vi "CRYCal Harmonics.vi"(0 "HT Option":bool[](array[boolean]), 1 "x":dbl[](array[numeric]), 2 "z":dbl[](array[numeric]), 3 "Index":i32, 5 "Method":u16, 7 "Harmonic":dbl[](array[numeric]), 9 "Freq resp curves":dbl[][](array[numeric]), 11 "Total Noise":dbl[](array[numeric]), 12 "Fs":dbl format="%.2f", 13 "max value1":dbl, 14 "max value2":dbl) -> (4 "Harmonic Track Out":T1(array[cluster]))   [LabVIEW 2013]
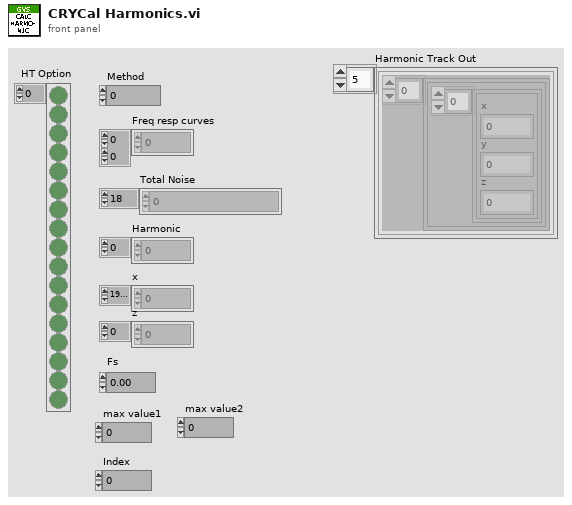
[diagram p1: front panel]
types:
  T1 = cluster{cluster{cluster{"x":dbl, "y":dbl, "z":dbl}[]}[]}[]
  T2 = cluster{"Freq resp curves clipped":cluster{cluster{"x":dbl, "y":dbl, "z":dbl}[]}[]}[]
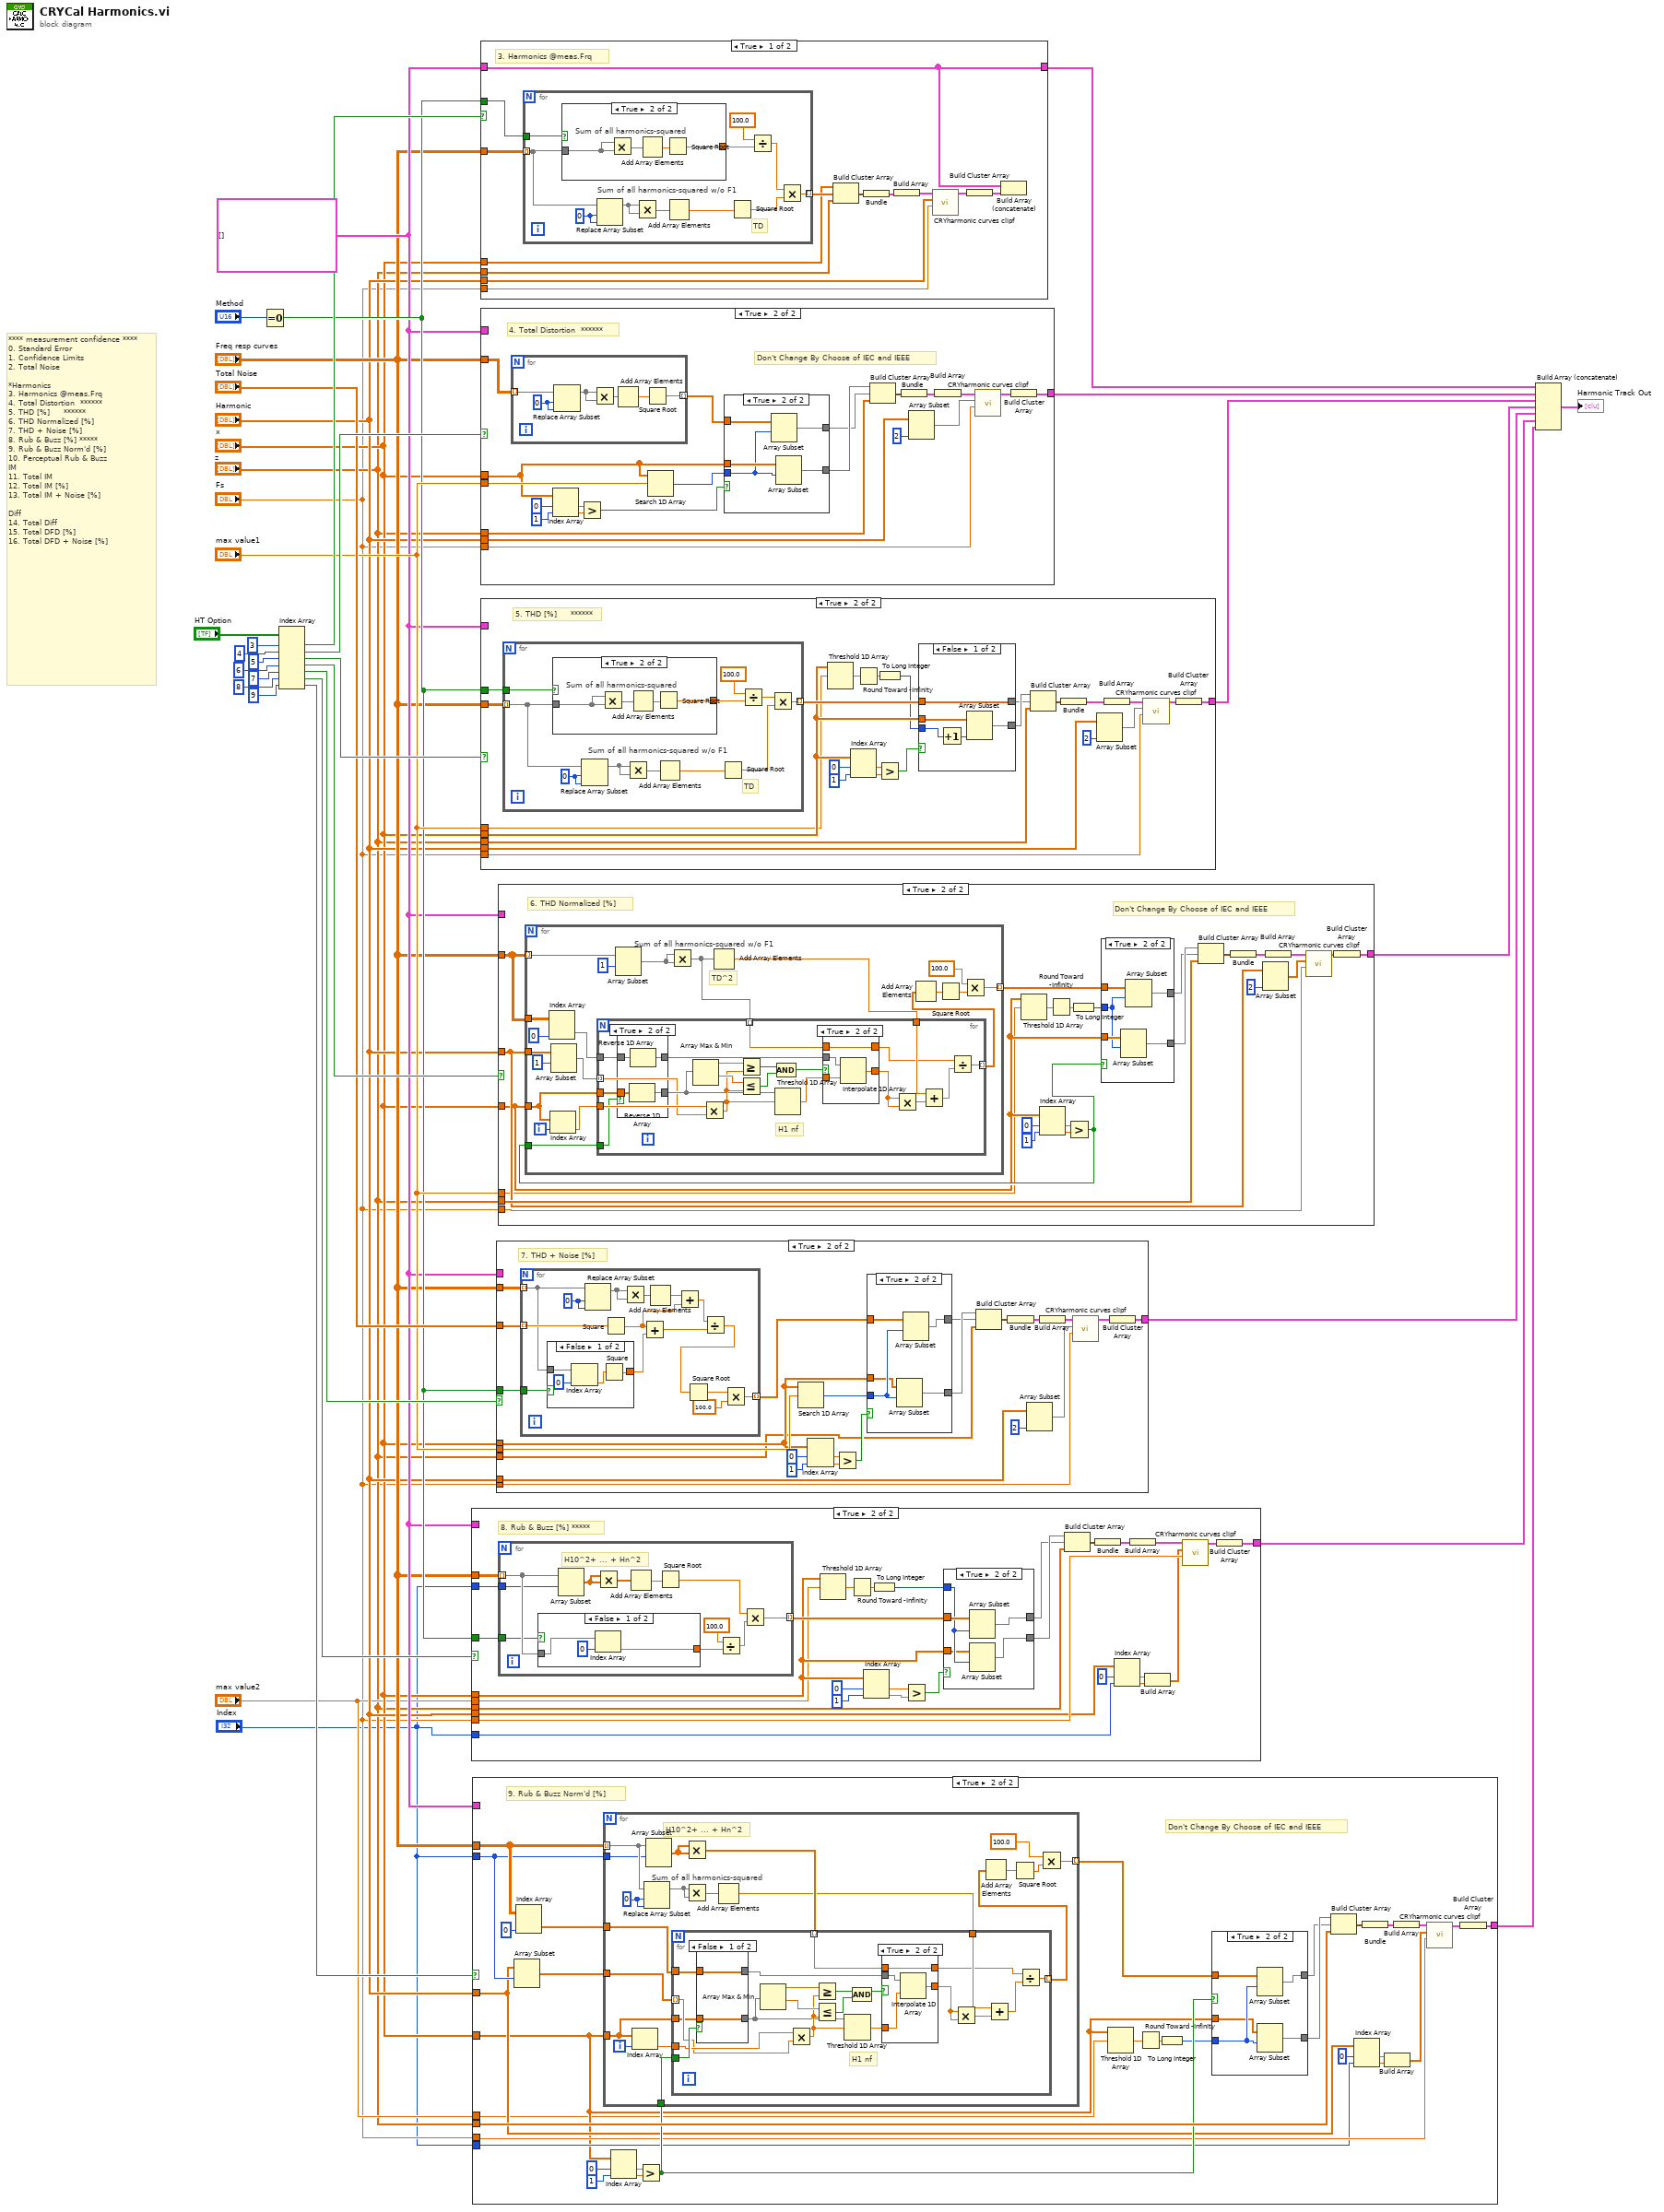
[diagram p0: block diagram]
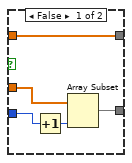
[diagram p3: hidden frame]
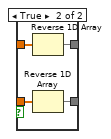
[diagram p4: hidden frame]
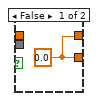
[diagram p5: hidden frame]
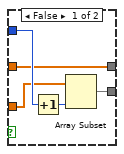
[diagram p7: hidden frame]
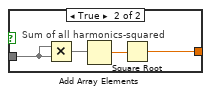
[diagram p8: hidden frame]
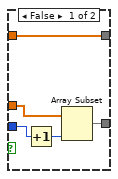
[diagram p10: hidden frame]
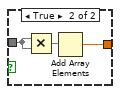
[diagram p11: hidden frame]
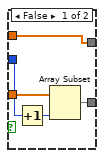
[diagram p13: hidden frame]
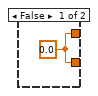
[diagram p15: hidden frame]
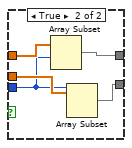
[diagram p17: hidden frame]
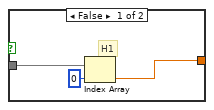
[diagram p18: hidden frame]
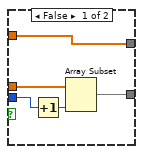
[diagram p20: hidden frame]
diagram:
  w10 = cluster{cluster{cluster[]}[]}[] []
  # "**** measurement confidence ****\n0. Standard Error\n1. Confidence Limits\n2. Total Noise\n\n*Harmonics\n3. Harmonics @meas.Frq\n4. Total Distortion  ******\n5. THD [%]     ******\n6. THD Normalized [%]\n7. THD + Noise [%]\n8. Rub & Buzz [%] *****\n9. Rub & Buzz Norm'd [%]\n10. Perceptual Rub & Buzz \nIM\n11. Total IM\n12. Total IM [%]\n13. Total IM + Noise [%]\n\nDiff\n14. Total Diff\n15. Total DFD [%]\n16. Total DFD + Noise [%]"
  n1 = Equal To 0?(x="Method") -> (x = 0?=w12:bool)
  n2 = Index Array(array="HT Option", index #1=3 ("index"), index #2=4 ("index"), index #3=5 ("index"), index #4=6 ("index"), index #5=7 ("index"), index #6=8 ("index"), index #7=9 ("index")) -> (element #1=w26:bool, element #2=w25:bool, element #3=w24:bool, element #4=w19:bool, element #5=w17:bool, element #6=w13:bool, element #7=w8:bool)
  n3 = case shown="True" w13 {
    tunnel: "Freq resp curves" -> [_ w58]
    tunnel: w12 -> [_ w57]
    tunnel: "x" -> [_ w39]
    tunnel: "max value2" -> [_ w38]
    tunnel: "Fs" -> [_ w56]
    tunnel: "z" -> [_ w55]
    tunnel: [w36 w49] -> w11
    tunnel: w10 -> [w36 _]
    tunnel: "Index" -> [_ w48]
    tunnel: "Harmonic" -> [_ w43]
    tunnel: "Index" -> [_ w42]
    frame False {
    }
    frame True {
      # "8. Rub & Buzz [%] *****"
      n4 = for {
        tunnel: [w81] -> w61 mode=indexing
        tunnel: w58 -> [w80] mode=indexing
        tunnel: w57 -> [w79]
        tunnel: w48 -> [w76]
        # "H10^2+ ... + Hn^2"
        n5 = case shown="False" w79 {
          tunnel: [w87 w92] -> w82
          tunnel: w80 -> [w88 w91]
          frame False {
            n6 = Index Array(array=w88, index=0) -> (element=w87:dbl)
          }
          frame True {
            # "Sum of all harmonics-squared"
            n7 = Multiply(x=w91, y=w91) -> (x*y=w90:dbl[])
            n8 = Add Array Elements(numeric array=w90) -> (sum=w93:dbl)
            n9 = Square Root(x=w93) -> (sqrt(x)=w92:dbl)
          }
        }
        n10 = Array Subset(array=w80, index=w76) -> (w78:dbl[])  [unwired: 1 in]
        n11 = Multiply(x=w78, y=w78) -> (x*y=w77:dbl[])
        n12 = Add Array Elements(numeric array=w77) -> (sum=w85:dbl)
        n13 = Square Root(x=w85) -> (sqrt(x)=w83:dbl)
        n14 = Divide(x=100.0, y=w82) -> (x/y=w84:dbl)
        n15 = Multiply(x=w83, y=w84) -> (x*y=w81:dbl)
      }
      n16 = Threshold 1D Array(2:w38, 3:w39) -> (0:w41:dbl)  [unwired: 1 in]
      n17 = Round Toward -Infinity(1:w41) -> (0:w40:dbl)
      n18 = Index Array(array=w39, index #1=0 ("index"), index #2=1 ("index")) -> (element #1=w52:dbl, element #2=w51:dbl)
      n19 = To Long Integer(number=w40) -> (32bit integer=w37:i32)
      n20 = Greater?(x=w52, y=w51) -> (0:w50:bool)
      n21 = case shown="True" w50 {
        tunnel: w37 -> [w70 w72]
        tunnel: [w68 w75] -> w62
        tunnel: [w67 w73] -> w60
        tunnel: w61 -> [w67 w74]
        tunnel: w39 -> [w66 w71]
        frame False {
          n22 = Increment(x=w70) -> (x+1=w69:i32)
          n23 = Array Subset(array=w66, length=w69) -> (w68:dbl[])  [unwired: 1 in]
        }
        frame True {
          n24 = Array Subset(array=w74, index=w72) -> (w73:dbl[])  [unwired: 1 in]
          n25 = Array Subset(array=w71, index=w72) -> (w75:dbl[])  [unwired: 1 in]
        }
      }
      n26 = Build Cluster Array(w62, w60, w55) -> (w64:cluster{"x":dbl, dbl, "Z":dbl}[])
      n27 = Bundle(w64) -> (w65:cluster{cluster{"x":dbl, dbl, "Z":dbl}[]})  [unwired: 1 in]
      n28 = Index Array(array=w43, index #1=0 ("Index"), index #2=w42) -> (element #1=w46:dbl, element #2=w45:dbl)
      n29 = Build Array(w65) -> (w59:cluster{cluster{"x":dbl, dbl, "Z":dbl}[]}[])
      n30 = Build Array(w46, w45) -> (w44:dbl[])
      n31 = call "CRYharmonic curves clipf.vi"("Fs"=w56, "Harmonics"=w44, "Freq resp curves"=w59) -> ("Freq resp curves clipped"=w63:cluster{cluster{"x":dbl, "y":dbl, "z":dbl}[]}[])  [unwired: 8 out]
      n32 = Build Cluster Array(w63) -> (w49:T2)
    }
  }
  n33 = case shown="True" w8 {
    tunnel: [w94 w118] -> w1
    tunnel: w10 -> [w94 _]
    tunnel: "Freq resp curves" -> [_ w104]
    tunnel: "Harmonic" -> [_ w101]
    tunnel: "x" -> [_ w97]
    tunnel: "max value2" -> [_ w96]
    tunnel: "z" -> [_ w113]
    tunnel: "Fs" -> [_ w107]
    tunnel: "Index" -> [_ w106]
    tunnel: "Index" -> [_ w102]
    frame False {
    }
    frame True {
      # "9. Rub & Buzz Norm'd [%]"
      # "Don't Change By Choose of IEC and IEEE"
      n34 = Array Subset(array=w101, index=w102) -> (w100:dbl[])  [unwired: 1 in]
      n35 = Index Array(array=w104, index (col)=0 ("disabled index (col)")) -> (element=w103:dbl[])  [unwired: 1 in]
      n36 = Index Array(array=w97, index #1=0 ("index"), index #2=1 ("index")) -> (element #1=w116:dbl, element #2=w117:dbl)
      n37 = Greater?(x=w116, y=w117) -> (0:w112:bool)
      n38 = for {
        tunnel: [w154] -> w121 mode=indexing
        tunnel: w104 -> [w142] mode=indexing
        tunnel: w97 -> [w140]
        tunnel: w112 -> [w141]
        tunnel: w102 -> [w138]
        tunnel: w103 -> [w137]
        tunnel: w100 -> [w136]
        i -> [w143]
        w145 = 0
        # "H10^2+ ... + Hn^2"
        # "Sum of all harmonics-squared"
        n39 = Index Array(array=w140, index=w143) -> (element=w153:dbl)
        n40 = Replace Array Subset(array=w142, new element=w145, index=w145) -> (w144:dbl[])
        n41 = Array Subset(array=w142, index=w138) -> (w139:dbl[])  [unwired: 1 in]
        n42 = Multiply(x=w139, y=w139) -> (x*y=w148:dbl[])
        n43 = Multiply(x=w144, y=w144) -> (x*y=w151:dbl[])
        n44 = Add Array Elements(numeric array=w151) -> (sum=w146:dbl)
        n45 = for {
          tunnel: w137 -> [w163]
          tunnel: w146 -> [w175]
          tunnel: w153 -> [w157]
          tunnel: w148 -> [w160] mode=indexing
          tunnel: [w171] -> w152 mode=indexing
          tunnel: w136 -> [w156] mode=indexing
          tunnel: w141 -> [w158]
          tunnel: w140 -> [w155]
          # "H1 nf"
          n46 = case shown="False" w158 {
            tunnel: w163 -> [w177 w178]
            tunnel: [w177 w181] -> w162
            tunnel: [w176 w180] -> w161
            tunnel: w155 -> [w176 w179]
            frame False {
            }
            frame True {
              n47 = Reverse 1D Array(array=w178) -> (reversed array=w181:dbl[])
              n48 = Reverse 1D Array(array=w179) -> (reversed array=w180:dbl[])
            }
          }
          n49 = Array Max & Min(array=w161) -> (max value=w168:dbl, min value=w167:dbl)  [unwired: 2 out]
          n50 = Multiply(x=w157, y=w156) -> (x*y=w166:dbl)
          n51 = Greater Or Equal?(x=w168, y=w166) -> (x >= y?=w169:bool)
          n52 = Less Or Equal?(x=w167, y=w166) -> (x <= y?=w164:bool)
          n53 = Threshold 1D Array(2:w166, 3:w161) -> (0:w170:dbl)  [unwired: 1 out]
          n54 = Compound Arithmetic op=AND(w169, w164) -> (w165:bool)
          n55 = case shown="True" w165 {
            tunnel: w162 -> [_ w183]
            tunnel: [w182 w184] -> w173
            tunnel: w170 -> [_ w185]
            tunnel: w160 -> [_ w186]
            tunnel: [w182 w186] -> w159
            frame False {
              w182 = 0.0 ("y")
            }
            frame True {
              n56 = Interpolate 1D Array(1:w185, 2:w183) -> (0:w184:dbl)
            }
          }
          n57 = Multiply(x=w173, y=w173) -> (x*y=w174:dbl)
          n58 = Add(x=w175, y=w174) -> (x+y=w172:dbl)
          n59 = Divide(x=w159, y=w172) -> (x/y=w171:dbl)
        }
        n60 = Add Array Elements(numeric array=w152) -> (sum=w149:dbl)
        n61 = Square Root(x=w149) -> (sqrt(x)=w147:dbl)
        n62 = Multiply(x=100.0, y=w147) -> (x*y=w154:dbl)
      }
      n63 = Threshold 1D Array(2:w96, 3:w97) -> (0:w98:dbl)  [unwired: 1 in]
      n64 = Round Toward -Infinity(1:w98) -> (0:w99:dbl)
      n65 = To Long Integer(number=w99) -> (32bit integer=w95:i32)
      n66 = case shown="True" w112 {
        tunnel: w95 -> [w130 w132]
        tunnel: [w128 w135] -> w122
        tunnel: w121 -> [w127 w134]
        tunnel: [w127 w133] -> w120
        tunnel: w97 -> [w126 w131]
        frame False {
          n67 = Increment(x=w130) -> (x+1=w129:i32)
          n68 = Array Subset(array=w126, length=w129) -> (w128:dbl[])  [unwired: 1 in]
        }
        frame True {
          n69 = Array Subset(array=w134, index=w132) -> (w133:dbl[])  [unwired: 1 in]
          n70 = Array Subset(array=w131, index=w132) -> (w135:dbl[])  [unwired: 1 in]
        }
      }
      n71 = Build Cluster Array(w122, w120, w113) -> (w124:cluster{"x":dbl, dbl, "Z":dbl}[])
      n72 = Index Array(array=w101, index #1=0 ("Index"), index #2=w106) -> (element #1=w110:dbl, element #2=w109:dbl)
      n73 = Bundle(w124) -> (w125:cluster{cluster{"x":dbl, dbl, "Z":dbl}[]})  [unwired: 1 in]
      n74 = Build Array(w110, w109) -> (w108:dbl[])
      n75 = Build Array(w125) -> (w119:cluster{cluster{"x":dbl, dbl, "Z":dbl}[]}[])
      n76 = call "CRYharmonic curves clipf.vi"("Fs"=w107, "Harmonics"=w108, "Freq resp curves"=w119) -> ("Freq resp curves clipped"=w123:cluster{cluster{"x":dbl, "y":dbl, "z":dbl}[]}[])  [unwired: 8 out]
      n77 = Build Cluster Array(w123) -> (w118:T2)
    }
  }
  n78 = case shown="True" w26 {
    tunnel: w10 -> [w192 w218]
    tunnel: "Freq resp curves" -> [w199 _]
    tunnel: [w192 w218] -> w23
    tunnel: w12 -> [w194 _]
    tunnel: "x" -> [w190 _]
    tunnel: "z" -> [w189 _]
    tunnel: "Harmonic" -> [w188 _]
    tunnel: "Fs" -> [w187 _]
    frame True {
      # "3. Harmonics @meas.Frq"
      n79 = for {
        tunnel: w199 -> [w201] mode=indexing
        tunnel: [w203] -> w198 mode=indexing
        tunnel: w194 -> [w200]
        w202 = 0
        # "TD"
        # "Sum of all harmonics-squared w/o F1"
        n80 = case shown="True" w200 {
          tunnel: [w211 w215] -> w204
          tunnel: w201 -> [w212 w214]
          frame False {
            # "H1"
            n81 = Index Array(array=w212, index=0) -> (element=w211:dbl)
          }
          frame True {
            # "Sum of all harmonics-squared"
            n82 = Multiply(x=w214, y=w214) -> (x*y=w217:dbl[])
            n83 = Add Array Elements(numeric array=w217) -> (sum=w216:dbl)
            n84 = Square Root(x=w216) -> (sqrt(x)=w215:dbl)
          }
        }
        n85 = Replace Array Subset(array=w201, new element=w202, index=w202) -> (w208:dbl[])
        n86 = Multiply(x=w208, y=w208) -> (x*y=w206:dbl[])
        n87 = Add Array Elements(numeric array=w206) -> (sum=w207:dbl)
        n88 = Square Root(x=w207) -> (sqrt(x)=w210:dbl)
        n89 = Divide(x=100.0, y=w204) -> (x/y=w205:dbl)
        n90 = Multiply(x=w205, y=w210) -> (x*y=w203:dbl)
      }
      n91 = Build Cluster Array(w190, w198, w189) -> (w195:cluster{"x":dbl, dbl, "Z":dbl}[])
      n92 = Bundle(w195) -> (w196:cluster{cluster{"x":dbl, dbl, "Z":dbl}[]})  [unwired: 1 in]
      n93 = Build Array(w196) -> (w197:cluster{cluster{"x":dbl, dbl, "Z":dbl}[]}[])
      n94 = call "CRYharmonic curves clipf.vi"("Fs"=w187, "Harmonics"=w188, "Freq resp curves"=w197) -> ("Freq resp curves clipped"=w191:cluster{cluster{"x":dbl, "y":dbl, "z":dbl}[]}[])  [unwired: 8 out]
      n95 = Build Cluster Array(w191) -> (w193:T2)
      n96 = Build Array (concatenate)(w192, w193) -> ()  [unwired: 1 out]
    }
    frame False {
    }
  }
  n97 = case shown="True" w25 {
    tunnel: w10 -> [w219 _]
    tunnel: "Freq resp curves" -> [_ w233]
    tunnel: "x" -> [_ w226]
    tunnel: "max value1" -> [_ w227]
    tunnel: "z" -> [_ w225]
    tunnel: "Harmonic" -> [_ w223]
    tunnel: "Fs" -> [_ w221]
    tunnel: [w219 w220] -> w22
    frame False {
    }
    frame True {
      # "4. Total Distortion  ******"
      # "Don't Change By Choose of IEC and IEEE"
      n98 = for {
        tunnel: w233 -> [w254] mode=indexing
        tunnel: [w252] -> w235 mode=indexing
        w255 = 0
        n99 = Replace Array Subset(array=w254, new element=w255, index=w255) -> (w257:dbl[])
        n100 = Multiply(x=w257, y=w257) -> (x*y=w256:dbl[])
        n101 = Add Array Elements(numeric array=w256) -> (sum=w253:dbl)
        n102 = Square Root(x=w253) -> (sqrt(x)=w252:dbl)
      }
      n103 = Index Array(array=w226, index #1=0 ("index"), index #2=1 ("index")) -> (element #1=w230:dbl, element #2=w229:dbl)
      n104 = Greater?(x=w230, y=w229) -> (0:w228:bool)
      n105 = Search 1D Array(1D array=w226, element=w227) -> (index of element=w237:i32)  [unwired: 1 in]
      n106 = case shown="True" w228 {
        tunnel: w237 -> [w246 w247]
        tunnel: w226 -> [w244 w251]
        tunnel: [w243 w250] -> w236
        tunnel: w235 -> [w242 w249]
        tunnel: [w242 w248] -> w234
        frame False {
          n107 = Increment(x=w246) -> (x+1=w245:i32)
          n108 = Array Subset(array=w244, length=w245) -> (w243:dbl[])  [unwired: 1 in]
        }
        frame True {
          n109 = Array Subset(array=w249, index=w247) -> (w248:dbl[])  [unwired: 1 in]
          n110 = Array Subset(array=w251, index=w247) -> (w250:dbl[])  [unwired: 1 in]
        }
      }
      n111 = Build Cluster Array(w236, w234, w225) -> (w239:cluster{"x":dbl, dbl, "Z":dbl}[])
      n112 = Bundle(w239) -> (w240:cluster{cluster{"x":dbl, dbl, "Z":dbl}[]})  [unwired: 1 in]
      n113 = Array Subset(array=w223, length=2 ("Array Length")) -> (w222:dbl[])  [unwired: 1 in]
      n114 = Build Array(w240) -> (w241:cluster{cluster{"x":dbl, dbl, "Z":dbl}[]}[])
      n115 = call "CRYharmonic curves clipf.vi"("Fs"=w221, "Harmonics"=w222, "Freq resp curves"=w241) -> ("Freq resp curves clipped"=w238:cluster{cluster{"x":dbl, "y":dbl, "z":dbl}[]}[])  [unwired: 8 out]
      n116 = Build Cluster Array(w238) -> (w220:T2)
    }
  }
  n117 = case shown="True" w24 {
    tunnel: w10 -> [w258 _]
    tunnel: [w258 w276] -> w21
    tunnel: "Freq resp curves" -> [_ w275]
    tunnel: w12 -> [_ w274]
    tunnel: "x" -> [_ w261]
    tunnel: "max value1" -> [_ w260]
    tunnel: "z" -> [_ w268]
    tunnel: "Harmonic" -> [_ w266]
    tunnel: "Fs" -> [_ w264]
    frame False {
    }
    frame True {
      # "5. THD [%]     ******"
      n118 = for {
        tunnel: w275 -> [w294] mode=indexing
        tunnel: [w297] -> w278 mode=indexing
        tunnel: w274 -> [w295]
        w296 = 0
        # "TD"
        # "Sum of all harmonics-squared w/o F1"
        n119 = case shown="True" w295 {
          tunnel: [w305 w309] -> w298
          tunnel: w294 -> [w306 w308]
          frame False {
            # "H1"
            n120 = Index Array(array=w306, index=0) -> (element=w305:dbl)
          }
          frame True {
            # "Sum of all harmonics-squared"
            n121 = Multiply(x=w308, y=w308) -> (x*y=w311:dbl[])
            n122 = Add Array Elements(numeric array=w311) -> (sum=w310:dbl)
            n123 = Square Root(x=w310) -> (sqrt(x)=w309:dbl)
          }
        }
        n124 = Replace Array Subset(array=w294, new element=w296, index=w296) -> (w302:dbl[])
        n125 = Multiply(x=w302, y=w302) -> (x*y=w300:dbl[])
        n126 = Add Array Elements(numeric array=w300) -> (sum=w301:dbl)
        n127 = Square Root(x=w301) -> (sqrt(x)=w304:dbl)
        n128 = Divide(x=100.0, y=w298) -> (x/y=w299:dbl)
        n129 = Multiply(x=w299, y=w304) -> (x*y=w297:dbl)
      }
      n130 = Threshold 1D Array(2:w260, 3:w261) -> (0:w263:dbl)  [unwired: 1 in]
      n131 = Index Array(array=w261, index #1=0 ("index"), index #2=1 ("index")) -> (element #1=w272:dbl, element #2=w273:dbl)
      n132 = Round Toward -Infinity(1:w263) -> (0:w262:dbl)
      n133 = To Long Integer(number=w262) -> (32bit integer=w259:i32)
      n134 = Greater?(x=w272, y=w273) -> (0:w269:bool)
      n135 = case shown="False" w269 {
        tunnel: w261 -> [w288 w293]
        tunnel: [w287 w292] -> w279
        tunnel: w259 -> [w286 w289]
        tunnel: w278 -> [w284 w291]
        tunnel: [w284 w290] -> w277
        frame False {
          n136 = Increment(x=w286) -> (x+1=w285:i32)
          n137 = Array Subset(array=w288, length=w285) -> (w287:dbl[])  [unwired: 1 in]
        }
        frame True {
          n138 = Array Subset(array=w291, index=w289) -> (w290:dbl[])  [unwired: 1 in]
          n139 = Array Subset(array=w293, index=w289) -> (w292:dbl[])  [unwired: 1 in]
        }
      }
      n140 = Build Cluster Array(w279, w277, w268) -> (w281:cluster{"x":dbl, dbl, "Z":dbl}[])
      n141 = Bundle(w281) -> (w282:cluster{cluster{"x":dbl, dbl, "Z":dbl}[]})  [unwired: 1 in]
      n142 = Array Subset(array=w266, length=2 ("Array Length")) -> (w265:dbl[])  [unwired: 1 in]
      n143 = Build Array(w282) -> (w283:cluster{cluster{"x":dbl, dbl, "Z":dbl}[]}[])
      n144 = call "CRYharmonic curves clipf.vi"("Fs"=w264, "Harmonics"=w265, "Freq resp curves"=w283) -> ("Freq resp curves clipped"=w280:cluster{cluster{"x":dbl, "y":dbl, "z":dbl}[]}[])  [unwired: 8 out]
      n145 = Build Cluster Array(w280) -> (w276:T2)
    }
  }
  n146 = case shown="True" w17 {
    tunnel: [w312 w329] -> w16
    tunnel: w10 -> [w312 _]
    tunnel: "Freq resp curves" -> [_ w328]
    tunnel: "Total Noise" -> [_ w327]
    tunnel: w12 -> [_ w326]
    tunnel: "x" -> [_ w320]
    tunnel: "max value1" -> [_ w325]
    tunnel: "z" -> [_ w318]
    tunnel: "Fs" -> [_ w314]
    tunnel: "Harmonic" -> [_ w313]
    frame False {
    }
    frame True {
      # "7. THD + Noise [%]"
      n147 = for {
        tunnel: [w352] -> w331 mode=indexing
        tunnel: w328 -> [w348] mode=indexing
        tunnel: w327 -> [w349] mode=indexing
        tunnel: w326 -> [w347]
        w359 = 0
        n148 = case shown="False" w347 {
          tunnel: [w364 w368] -> w357
          tunnel: w348 -> [w363 w367]
          frame False {
            n149 = Index Array(array=w363, index=0) -> (element=w362:dbl)
            n150 = Square(x=w362) -> (x^2=w364:dbl)
          }
          frame True {
            n151 = Multiply(x=w367, y=w367) -> (x*y=w366:dbl[])
            n152 = Add Array Elements(numeric array=w366) -> (sum=w368:dbl)
          }
        }
        n153 = Replace Array Subset(array=w348, new element=w359, index=w359) -> (w361:dbl[])
        n154 = Square(x=w349) -> (x^2=w353:dbl)
        n155 = Multiply(x=w361, y=w361) -> (x*y=w360:dbl[])
        n156 = Add(x=w353, y=w357) -> (x+y=w355:dbl)
        n157 = Add Array Elements(numeric array=w360) -> (sum=w358:dbl)
        n158 = Add(x=w358, y=w353) -> (x+y=w356:dbl)
        n159 = Divide(x=w356, y=w355) -> (x/y=w354:dbl)
        n160 = Square Root(x=w354) -> (sqrt(x)=w351:dbl)
        n161 = Multiply(x=w351, y=100.0) -> (x*y=w352:dbl)
      }
      n162 = Search 1D Array(1D array=w320, element=w325) -> (index of element=w333:i32)  [unwired: 1 in]
      n163 = Index Array(array=w320, index #1=0 ("index"), index #2=1 ("index")) -> (element #1=w323:dbl, element #2=w324:dbl)
      n164 = Greater?(x=w323, y=w324) -> (0:w319:bool)
      n165 = case shown="True" w319 {
        tunnel: w333 -> [w341 w343]
        tunnel: [w339 w346] -> w332
        tunnel: w331 -> [w338 w345]
        tunnel: [w338 w344] -> w330
        tunnel: w320 -> [w337 w342]
        frame False {
          n166 = Increment(x=w341) -> (x+1=w340:i32)
          n167 = Array Subset(array=w337, length=w340) -> (w339:dbl[])  [unwired: 1 in]
        }
        frame True {
          n168 = Array Subset(array=w342, index=w343) -> (w346:dbl[])  [unwired: 1 in]
          n169 = Array Subset(array=w345, index=w343) -> (w344:dbl[])  [unwired: 1 in]
        }
      }
      n170 = Build Cluster Array(w332, w330, w318) -> (w335:cluster{"x":dbl, dbl, "Z":dbl}[])
      n171 = Bundle(w335) -> (w336:cluster{cluster{"x":dbl, dbl, "Z":dbl}[]})  [unwired: 1 in]
      n172 = Array Subset(array=w313, length=2 ("Array Length")) -> (w315:dbl[])  [unwired: 1 in]
      n173 = Build Array(w336) -> (w317:cluster{cluster{"x":dbl, dbl, "Z":dbl}[]}[])
      n174 = call "CRYharmonic curves clipf.vi"("Fs"=w314, "Harmonics"=w315, "Freq resp curves"=w317) -> ("Freq resp curves clipped"=w334:cluster{cluster{"x":dbl, "y":dbl, "z":dbl}[]}[])  [unwired: 8 out]
      n175 = Build Cluster Array(w334) -> (w329:T2)
    }
  }
  n176 = case shown="True" w19 {
    tunnel: "Freq resp curves" -> [_ w386]
    tunnel: "Harmonic" -> [_ w377]
    tunnel: "x" -> [_ w372]
    tunnel: "Fs" -> [_ w380]
    tunnel: "max value1" -> [_ w371]
    tunnel: "z" -> [_ w379]
    tunnel: [w369 w375] -> w18
    tunnel: w10 -> [w369 _]
    frame False {
    }
    frame True {
      # "6. THD Normalized [%]"
      # "Don't Change By Choose of IEC and IEEE"
      n177 = Threshold 1D Array(2:w371, 3:w372) -> (0:w373:dbl)  [unwired: 1 in]
      n178 = Index Array(array=w372, index #1=0 ("index"), index #2=1 ("index")) -> (element #1=w383:dbl, element #2=w382:dbl)
      n179 = Round Toward -Infinity(1:w373) -> (0:w374:dbl)
      n180 = Greater?(x=w383, y=w382) -> (0:w381:bool)
      n181 = for {
        tunnel: w386 -> [w406] mode=indexing
        tunnel: [w412] -> w388 mode=indexing
        tunnel: w386 -> [w423]
        tunnel: w372 -> [w419]
        tunnel: w381 -> [w410]
        tunnel: w377 -> [w409]
        i -> [w417]
        # "TD^2"
        # "Sum of all harmonics-squared w/o F1"
        n182 = Index Array(array=w423, index (col)=0 ("disabled index (col)")) -> (element=w421:dbl[])  [unwired: 1 in]
        n183 = Index Array(array=w419, index=w417) -> (element=w418:dbl)
        n184 = Array Subset(array=w409, index=1) -> (w407:dbl[])  [unwired: 1 in]
        n185 = Array Subset(array=w406, index=1) -> (w404:dbl[])  [unwired: 1 in]
        n186 = Multiply(x=w404, y=w404) -> (x*y=w414:dbl[])
        n187 = Add Array Elements(numeric array=w414) -> (sum=w420:dbl)
        n188 = for {
          tunnel: w421 -> [w426]
          tunnel: w420 -> [w444]
          tunnel: w419 -> [w429]
          tunnel: w418 -> [w441]
          tunnel: w414 -> [w431] mode=indexing
          tunnel: [w438] -> w416 mode=indexing
          tunnel: w410 -> [w427]
          tunnel: w407 -> [w424] mode=indexing
          # "H1 nf"
          n189 = case shown="True" w427 {
            tunnel: w429 -> [w446 w450]
            tunnel: [w446 w449] -> w428
            tunnel: w426 -> [w445 w448]
            tunnel: [w445 w447] -> w425
            frame False {
            }
            frame True {
              n190 = Reverse 1D Array(array=w450) -> (reversed array=w449:dbl[])
              n191 = Reverse 1D Array(array=w448) -> (reversed array=w447:dbl[])
            }
          }
          n192 = Array Max & Min(array=w428) -> (max value=w437:dbl, min value=w436:dbl)  [unwired: 2 out]
          n193 = Multiply(x=w441, y=w424) -> (x*y=w435:dbl)
          n194 = Greater Or Equal?(x=w437, y=w435) -> (x >= y?=w433:bool)
          n195 = Less Or Equal?(x=w436, y=w435) -> (x <= y?=w432:bool)
          n196 = Threshold 1D Array(2:w435, 3:w428) -> (0:w443:dbl)  [unwired: 1 out]
          n197 = Compound Arithmetic op=AND(w433, w432) -> (w434:bool)
          n198 = case shown="True" w434 {
            tunnel: w425 -> [_ w454]
            tunnel: w443 -> [_ w453]
            tunnel: [w451 w452] -> w440
            tunnel: w431 -> [_ w455]
            tunnel: [w451 w455] -> w430
            frame False {
              w451 = 0.0 ("y")
            }
            frame True {
              n199 = Interpolate 1D Array(1:w453, 2:w454) -> (0:w452:dbl)
            }
          }
          n200 = Multiply(x=w440, y=w440) -> (x*y=w442:dbl)
          n201 = Add(x=w444, y=w442) -> (x+y=w439:dbl)
          n202 = Divide(x=w430, y=w439) -> (x/y=w438:dbl)
        }
        n203 = Add Array Elements(numeric array=w416) -> (sum=w415:dbl)
        n204 = Square Root(x=w415) -> (sqrt(x)=w413:dbl)
        n205 = Multiply(x=100.0, y=w413) -> (x*y=w412:dbl)
      }
      n206 = To Long Integer(number=w374) -> (32bit integer=w370:i32)
      n207 = case shown="True" w381 {
        tunnel: w370 -> [w398 w400]
        tunnel: w372 -> [w396 w403]
        tunnel: [w395 w402] -> w389
        tunnel: w388 -> [w394 w401]
        tunnel: [w394 w399] -> w387
        frame False {
          n208 = Increment(x=w398) -> (x+1=w397:i32)
          n209 = Array Subset(array=w396, length=w397) -> (w395:dbl[])  [unwired: 1 in]
        }
        frame True {
          n210 = Array Subset(array=w403, index=w400) -> (w402:dbl[])  [unwired: 1 in]
          n211 = Array Subset(array=w401, index=w400) -> (w399:dbl[])  [unwired: 1 in]
        }
      }
      n212 = Build Cluster Array(w389, w387, w379) -> (w391:cluster{"x":dbl, dbl, "Z":dbl}[])
      n213 = Bundle(w391) -> (w392:cluster{cluster{"x":dbl, dbl, "Z":dbl}[]})  [unwired: 1 in]
      n214 = Array Subset(array=w377, length=2 ("Array Length")) -> (w376:dbl[])  [unwired: 1 in]
      n215 = Build Array(w392) -> (w393:cluster{cluster{"x":dbl, dbl, "Z":dbl}[]}[])
      n216 = call "CRYharmonic curves clipf.vi"("Fs"=w380, "Harmonics"=w376, "Freq resp curves"=w393) -> ("Freq resp curves clipped"=w390:cluster{cluster{"x":dbl, "y":dbl, "z":dbl}[]}[])  [unwired: 8 out]
      n217 = Build Cluster Array(w390) -> (w375:T2)
    }
  }
  n218 = Build Array (concatenate)(w23, w22, w21, w18, w16, w11, w1) -> (→"Harmonic Track Out":T2)
